vi "Array_Erd_Data_Erd_Id.vi"(5 "ERD Data Out out":T1[](array[typedef]) {"ERD Number" format="%.0x"}) -> (8 "Array_Erd_Number":string[](array[string]), 10 "Array_Erd_Data":string[](array[string]))   [LabVIEW 2023]
uses:
  Common/LabVIEW GEA2 Toolkit/GEA3/type defs/ERD Read Data Out.ctl
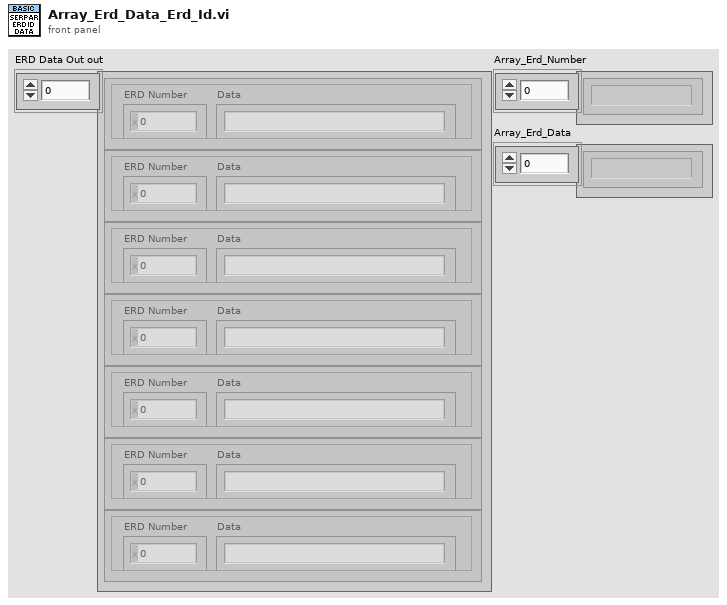
[diagram p1: front panel]
types:
  T1 = typedef "ERD Read Data Out.ctl" = cluster{"ERD Number":u16, "Data":string}
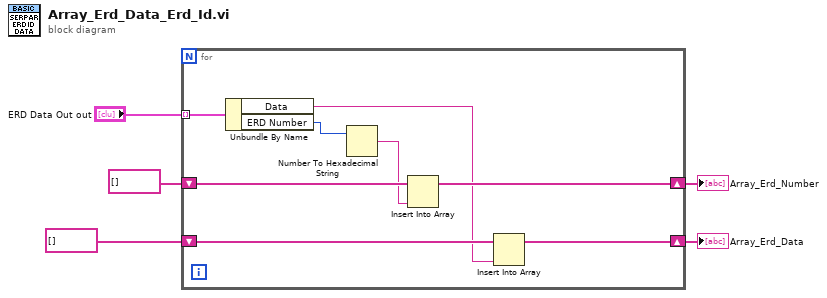
[diagram p0: block diagram]
diagram:
  n1 = for {
    tunnel: "ERD Data Out out" -> [w13] mode=indexing
    shift-right: [w10] -> w2
    shift-left: string[] [] -> [w11]
    shift-right: [w8] -> w1
    shift-left: string[] [] -> [w7]
    n2 = Unbundle By Name(w13) -> ("Data"=w6:string, "ERD Number"=w12:u16)
    n3 = Number To Hexadecimal String(2:w12) -> (0:w9:string)  [unwired: 1 in]
    n4 = Insert Into Array(array=w11, new element=w9) -> (w10:string[])  [unwired: 1 in]
    n5 = Insert Into Array(array=w7, new element=w6) -> (w8:string[])  [unwired: 1 in]
  }
  "Array_Erd_Number" <- w2
  "Array_Erd_Data" <- w1
